vi "ReadGroup.vi"(7 "LabVIEW Web Service Request":refnum<class "Web Request.lvclass">, 11 "groupName":T1) -> ()   [LabVIEW 2013]
uses:
  <vilib>/wsapi/Web Request.lvclass
  <vilib>/NI/TagWebClient/API/String Controls/groupName.ctl
  <vilib>/NI/TagWebClient/API/JSON Formats/ReadGroup Results.ctl
  <vilib>/NI/TagWebClient/API/Logical Groups/Values.ctl
  <vilib>/NI/TagWebClient/API/String Controls/value.ctl
  <vilib>/NI/TagWebClient/API/tagweb client API.lvlib
panel:
  # "Use the Web Service Request input terminal to call the VIs on the Web Services palette. Do not remove it from the connector pane unless you don't need access to the palette."
  # "Each additional control wired to the connector pane will be available as an input in the URL. To include an indicator in terminal-mode output (the default setting), it must also be wired to the connector pane."
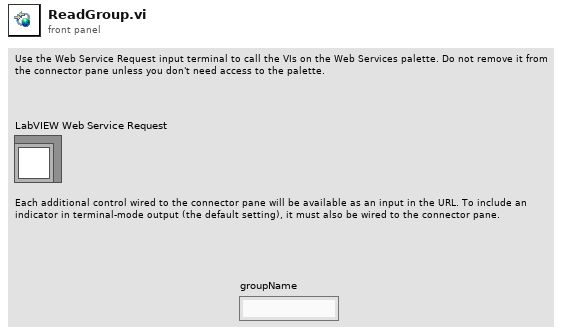
[diagram p1: front panel]
types:
  T1 = typedef "tagweb client API.lvlib/groupName.ctl" = string
  T2 = typedef "tagweb client API.lvlib/ReadGroup Results.ctl" = cluster{"Values":T3}
  T3 = typedef "tagweb client API.lvlib/Values.ctl" = T4[]
  T4 = typedef "tagweb client API.lvlib/value.ctl" = string
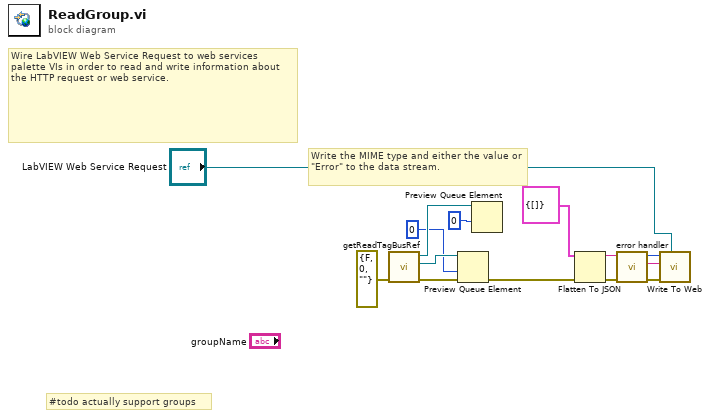
[diagram p0: block diagram]
diagram:
  # "#todo actually support groups"
  # "Write the MIME type and either the value or \"Error\" to the data stream."
  # "Wire LabVIEW Web Service Request to web services palette VIs in order to read and write information about the HTTP request or web service."
  n1 = call "getReadTagBusRef.vi"("error in (no error)"=errorcluster {"status"=FALSE, "code"=0, "source"=""}) -> ("error out"=w14:errorcluster, "read data table"=w13:refnum<queue>, "read data dictionary"=w11:refnum<queue>)  [unwired: 7 in, 1 out]
  n2 = Preview Queue Element(queue=w13, timeout in ms (-1)=0, error in (no error)=w14) -> (error out=w10:errorcluster)  [unwired: 3 out]
  n3 = Preview Queue Element(queue=w11, timeout in ms (-1)=0) -> ()  [unwired: 1 in, 4 out]
  n4 = Flatten To JSON(anything=T2 {"Values"=[]} ("Read Group Results"), error in (no error)=w10) -> (JSON string=w8:string, 11:w9:errorcluster)  [unwired: 1 in]
  n5 = call "error handler.vi"("error in (no error)"=w9, "Success Message"=w8) -> ("error out"=w5:errorcluster, "Response String"=w6:string, "Response Code"=w7:i32)  [unwired: 7 in]
  n6 = call <vilib>:"Write To Web.vi"("Web Request in"="LabVIEW Web Service Request", "error in (no error)"=w5, "Response String"=w6, "Response Code"=w7) -> ()  [unwired: 7 in, 1 out]
